vi "UI Parser (SubVI).vi"(0 "DATA INPUT":dbl[](array[numeric])) -> (4 "LC Array":dbl[](array[numeric]), 6 "PT Array":dbl[](array[numeric]), 8 "TC Array":dbl[](array[numeric]), 10 "LS Array":dbl[](array[numeric]), 14 "Valves":dbl[](array[numeric]), 15 "GO's":dbl[](array[numeric]))   [LabVIEW 2020]
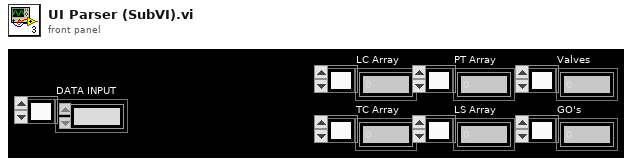
[diagram p1: front panel]
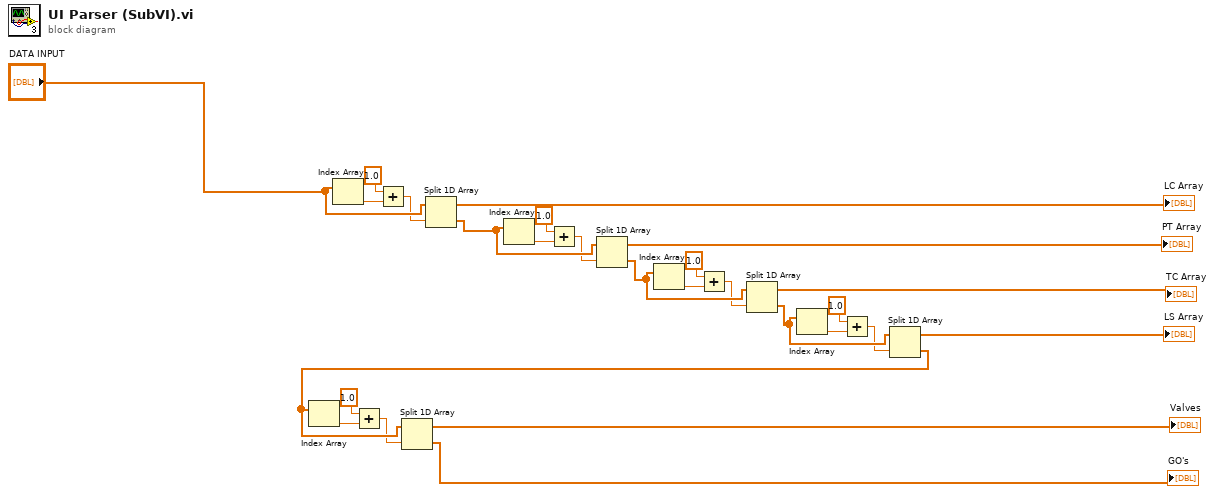
[diagram p0: block diagram]
diagram:
  n1 = Index Array(array="DATA INPUT") -> (element=w6:dbl)  [unwired: 1 in]
  n2 = Add(x=1.0, y=w6) -> (x+y=w5:dbl)
  n3 = Split 1D Array(array="DATA INPUT", index=w5) -> (first subarray=→"LC Array":dbl[], second subarray=w19:dbl[])
  n4 = Index Array(array=w19) -> (element=w7:dbl)  [unwired: 1 in]
  n5 = Add(x=1.0, y=w7) -> (x+y=w8:dbl)
  n6 = Split 1D Array(array=w19, index=w8) -> (first subarray=→"PT Array":dbl[], second subarray=w20:dbl[])
  n7 = Index Array(array=w20) -> (element=w10:dbl)  [unwired: 1 in]
  n8 = Add(x=1.0, y=w10) -> (x+y=w11:dbl)
  n9 = Split 1D Array(array=w20, index=w11) -> (first subarray=→"TC Array":dbl[], second subarray=w21:dbl[])
  n10 = Index Array(array=w21) -> (element=w13:dbl)  [unwired: 1 in]
  n11 = Add(x=1.0, y=w13) -> (x+y=w14:dbl)
  n12 = Split 1D Array(array=w21, index=w14) -> (first subarray=→"LS Array":dbl[], second subarray=w22:dbl[])
  n13 = Index Array(array=w22) -> (element=w16:dbl)  [unwired: 1 in]
  n14 = Add(x=1.0, y=w16) -> (x+y=w17:dbl)
  n15 = Split 1D Array(array=w22, index=w17) -> (first subarray=→"Valves":dbl[], second subarray=→"GO's":dbl[])
